vi "Change Joystick Values.vi"(1 "Change -1 to?":dbl, 2 "Change 1 to?":dbl, 3 "Joystick Input":dbl(slide) scale=-1.0..1.0) -> (0 "Output Value":dbl)   [LabVIEW 2011]
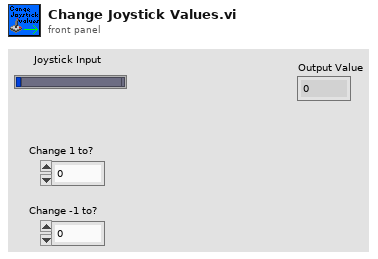
[diagram p1: front panel]
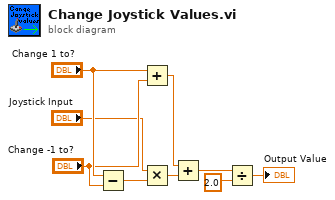
[diagram p0: block diagram]
diagram:
  n1 = Subtract(x="Change 1 to?", y="Change -1 to?") -> (x-y=w7:dbl)
  n2 = Add(x="Change 1 to?", y="Change -1 to?") -> (x+y=w4:dbl)
  n3 = Multiply(x="Joystick Input", y=w7) -> (x*y=w5:dbl)
  n4 = Add(x=w4, y=w5) -> (x+y=w2:dbl)
  n5 = Divide(x=w2, y=2.0) -> (x/y=→"Output Value":dbl)
